vi "DFConfig Indexer.vi"(8 "error in (no error)":errorcluster, 9 "Datafinder Indexer":T1={"repeat"=enum."daily", "enable_observer"=TRUE, "starttime"=timestamp(0 s since 1904-01-01), "timeout"=30000}, 10 "CrawlSettings ID (\"\")":string, 11 "My.DataFinder In":string) -> (0 "error out":errorcluster, 3 "My.DataFinder Out":string)   [LabVIEW 2011]
uses:
  DFConfig INDEXER.ctl
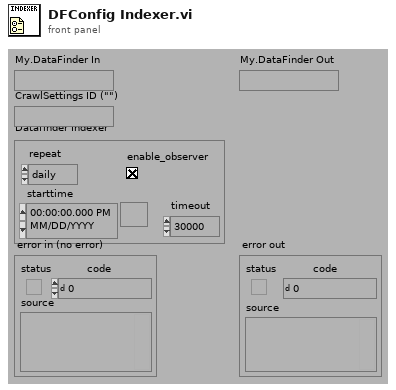
[diagram p1: front panel]
types:
  T1 = typedef "DFConfig INDEXER.ctl" = cluster{"repeat":enum16{"hourly", "daily", "weekly", "never"}, "enable_observer":bool, "starttime":timestamp, "timeout":i32}
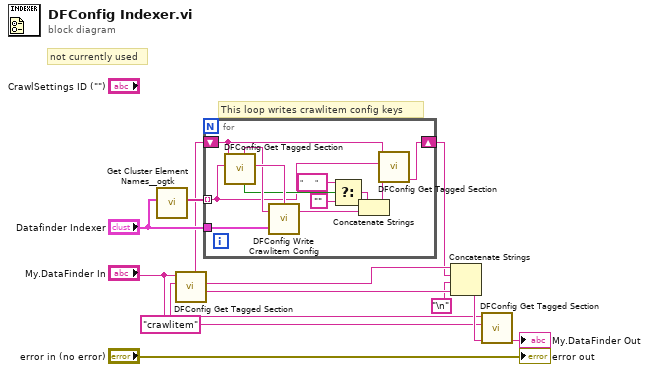
[diagram p0: block diagram]
diagram:
  w2 = "crawlitem"
  # "This loop writes crawlitem config keys"
  # "not currently used"
  n1 = call "Get Cluster Element Names__ogtk.vi"("Cluster"="Datafinder Indexer") -> ("Element Names"=w6:string[])  [unwired: 1 in, 9 out]
  n2 = call "DFConfig Get Tagged Section.vi"("Tag (\"\")"=w2, "String"="My.DataFinder In") -> ("End Tag"=w12:string, "Start Tag"=w7:string, "InnerString"=w4:string)  [unwired: 1 in, 6 out]
  n3 = for {
    tunnel: w6 -> [w16] mode=indexing
    shift-right: [w20] -> w3
    shift-left: w4 -> [w21]
    tunnel: "Datafinder Indexer" -> [w23]
    n4 = call "DFConfig Get Tagged Section.vi"("Tag (\"\")"=w16, "String"=w21) -> ("Start Tag"=w24:string, "Not Found?"=w17:bool, "InnerString"=w22:string)  [unwired: 1 in, 6 out]
    n5 = call "DFConfig Write Crawlitem Config.vi"("Datafinder Indexer"=w23, "Config In"=w22, "Tag (\"\")"=w24) -> ("Config Out"=w19:string)  [unwired: 2 out]
    n6 = Select(t="      ", s=w17, f="") -> (s? t:f=w13:string)
    n7 = Concatenate Strings(w13, w19) -> (w18:string)
    n8 = call "DFConfig Get Tagged Section.vi"("Replacement String (\"\")"=w18, "Tag (\"\")"=w16, "String"=w21) -> ("String with Replacement"=w20:string)  [unwired: 8 out]
  }
  n9 = Concatenate Strings(w7, w3, "\n", w12) -> (w11:string)
  n10 = call "DFConfig Get Tagged Section.vi"("Replacement String (\"\")"=w11, "Tag (\"\")"=w2, "String"="My.DataFinder In") -> ("String with Replacement"=→"My.DataFinder Out":string)  [unwired: 8 out]
  "error out" <- "error in (no error)"
